vi "Glimpse fill time table with evenly spaced times.vi"(3 "Element 0 of TTB":u32, 4 "Number of frames in sequence":i32, 5 "Milliseconds per frame":dbl format="%.2f") -> (0 "Sequence Range":cluster{i32, i32}, 1 "Time  per frame":dbl format="%.2f", 2 "TTB Array":u32[](array[numeric]))   [LabVIEW 2016]
doc: "To be called after a high-speed video acquisition is completed; properly fills the time table array and other globals."
panel:
  in  "Milliseconds per frame":dbl format="%.2f"
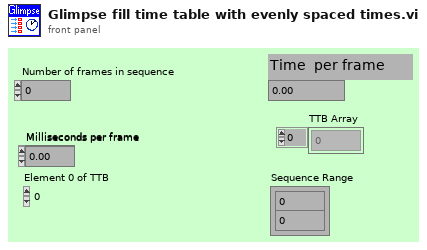
[diagram p1: front panel]
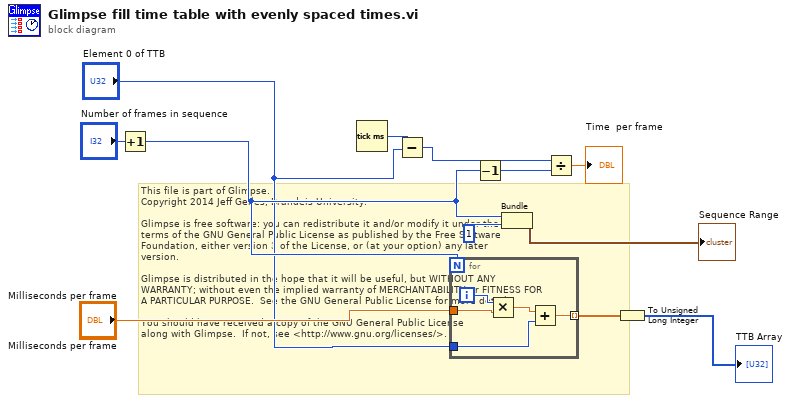
[diagram p0: block diagram]
diagram:
  # "This file is part of Glimpse. \nCopyright 2014 Jeff Gelles, Brandeis University.    \n\nGlimpse is free software: you can redistribute it and/or modify it under the \nterms of the GNU General Public License as published by the Free Software \nFoundation, either version 3 of the License, or (at your option) any later \nversion.\n\nGlimpse is distributed in the hope that it will be useful, but WITHOUT ANY \nWARRANTY; without even the implied warranty of MERCHANTABILITY or FITNESS FOR \nA PARTICULAR PURPOSE.  See the GNU General Public License for more details.\n\nYou should have received a copy of the GNU General Public License\nalong with Glimpse.  If not, see <http://www.gnu.org/licenses/>."
  n1 = Increment(x="Number of frames in sequence") -> (x+1=w12:i32)
  n2 = Tick Count (ms)() -> (millisecond timer value=w5:u32)
  n3 = Subtract(x=w5, y="Element 0 of TTB") -> (x-y=w6:u32)
  n4 = for {
    N: w12 -> [_]
    tunnel: "Milliseconds per frame" -> [w16]
    tunnel: "Element 0 of TTB" -> [w15]
    tunnel: [w13] -> w11 mode=indexing
    i -> [w17]
    n5 = Multiply(x=w17, y=w16) -> (x*y=w14:dbl)
    n6 = Add(x=w14, y=w15) -> (x+y=w13:dbl)
  }
  n7 = Decrement(x=w12) -> (x-1=w2:i32)
  n8 = Bundle(w12, 1) -> (→"Sequence Range":cluster{i32, i32})  [unwired: 1 out]
  n9 = Divide(x=w6, y=w2) -> (x/y=→"Time  per frame":dbl)
  n10 = To Unsigned Long Integer(number=w11) -> (unsigned 32bit integer=→"TTB Array":u32[])
